vi "RefStruct_CONVERT.vi"(1 "RefStruct":T12={"RefNormal"={"Mode"=0, "Fliter"=1, "AccCode"=0, "AccMask"=0, "kBaudRate"=0, "Timing0"=0, "Timing1"=0, "CANRX_EN"=0, "UARTBAUD"=0}, "Reserved"=0, "BaudType"={"Baud"=0, "SJW"=1, "BRP"=1, "SAM"=0, "PHSEG2_SEL"=0, "PRSEG"=1, "PHSEG1"=1, "PHSEG2"=1}} {"RefNormal"."kBaudRate" items=["SelfDefine", "5 kbps", "10 kbps", "20 kbps", "40 kbps", "50 kbps", "80 kbps", "100 kbps", "125 kbps", "200 kbps", "250 kbps", "400 kbps", "500 kbps", "666 kbps", "800 kbps", "1000 kbps", "33.33 kbps", "66.66 kbps", "83.33 kbps"]; "RefNormal"."AccMask" format="%x"; "RefNormal"."AccCode" format="%x"; "RefNormal"."Fliter" items=["接收所有类型"=1, "只接收标准帧"=2, "只接收扩展帧"=3]; "RefNormal"."Mode" items=["正常工作", "仅侦听模式", "自测模式（环回）"]; "BaudType"."PHSEG2" items=["CAN_BIT_1TQ"=1, "CAN_BIT_2TQ"=2, "CAN_BIT_3TQ"=3, "CAN_BIT_4TQ"=4, "CAN_BIT_5TQ"=5, "CAN_BIT_6TQ"=6, "CAN_BIT_7TQ"=7, "CAN_BIT_8TQ"=8]; "BaudType"."PHSEG1" items=["CAN_BIT_1TQ"=1, "CAN_BIT_2TQ"=2, "CAN_BIT_3TQ"=3, "CAN_BIT_4TQ"=4, "CAN_BIT_5TQ"=5, "CAN_BIT_6TQ"=6, "CAN_BIT_7TQ"=7, "CAN_BIT_8TQ"=8]; "BaudType"."PRSEG" items=["CAN_BIT_1TQ"=1, "CAN_BIT_2TQ"=2, "CAN_BIT_3TQ"=3, "CAN_BIT_4TQ"=4, "CAN_BIT_5TQ"=5, "CAN_BIT_6TQ"=6, "CAN_BIT_7TQ"=7, "CAN_BIT_8TQ"=8]; "BaudType"."PHSEG2_SEL" items=["由相位缓冲段1时间决定", "可编程"]; "BaudType"."SAM" items=["采样一次", "采样三次"]; "BaudType"."BRP" items=["1"=1, "2"=2, "3"=3, "4"=4, "5"=5, "6"=6, "7"=7, "8"=8, "9"=9, "10"=10, "11"=11, "12"=12, "13"=13, "14"=14, "15"=15, "16"=16, "17"=17, "18"=18, "19"=19, "20"=20, "21"=21, "22"=22, "23"=23, "24"=24, "25"=25, "26"=26, "27"=27, "28"=28, "29"=29, "30"=30, "31"=31, "32"=32, "33"=33, "34"=34, "35"=35, "36"=36, "37"=37, "38"=38, "39"=39, "40"=40, "41"=41, "42"=42, "43"=43, "44"=44, "45"=45, "46"=46, "47"=47, "48"=48, "49"=49, "50"=50, "51"=51, "52"=52, "53"=53, "54"=54, "55"=55, "56"=56, "57"=57, "58"=58, "59"=59, "60"=60, "61"=61, "62"=62, "63"=63, "64"=64]; "BaudType"."SJW" items=["1TQ"=1, "2TQ"=2, "3TQ"=3, "4TQ"=4]}) -> (0 "RefStruct_1":T1={"Mode"=0, "Fliter"=1, "ACR 0"=0, "ACR 1"=0, "ACR 2"=0, "ACR 3"=0, "AMR 0"=0, "AMR 1"=0, "AMR 2"=0, "AMR 3"=0, "kBaudRate"=0, "Timing 0"=0, "Timing 1"=0, "CANRX_EN"=0, "UARTBAUD"=0, "Reserved"=0, "Baud 0"=0, "Baud 1"=0, "Baud 2"=0, "Baud 3"=0, "SJW"=1, "BRP"=1, "SAM"=0, "PHSEG2_SEL"=0, "PRSEG"=1, "PHSEG1"=1, "PHSEG2"=1} {"PHSEG2" items=["CAN_BIT_1TQ"=1, "CAN_BIT_2TQ"=2, "CAN_BIT_3TQ"=3, "CAN_BIT_4TQ"=4, "CAN_BIT_5TQ"=5, "CAN_BIT_6TQ"=6, "CAN_BIT_7TQ"=7, "CAN_BIT_8TQ"=8]; "PHSEG1" items=["CAN_BIT_1TQ"=1, "CAN_BIT_2TQ"=2, "CAN_BIT_3TQ"=3, "CAN_BIT_4TQ"=4, "CAN_BIT_5TQ"=5, "CAN_BIT_6TQ"=6, "CAN_BIT_7TQ"=7, "CAN_BIT_8TQ"=8]; "PRSEG" items=["CAN_BIT_1TQ"=1, "CAN_BIT_2TQ"=2, "CAN_BIT_3TQ"=3, "CAN_BIT_4TQ"=4, "CAN_BIT_5TQ"=5, "CAN_BIT_6TQ"=6, "CAN_BIT_7TQ"=7, "CAN_BIT_8TQ"=8]; "PHSEG2_SEL" items=["由相位缓冲段1时间决定", "可编程"]; "SAM" items=["采样一次", "采样三次"]; "BRP" items=["1"=1, "2"=2, "3"=3, "4"=4, "5"=5, "6"=6, "7"=7, "8"=8, "9"=9, "10"=10, "11"=11, "12"=12, "13"=13, "14"=14, "15"=15, "16"=16, "17"=17, "18"=18, "19"=19, "20"=20, "21"=21, "22"=22, "23"=23, "24"=24, "25"=25, "26"=26, "27"=27, "28"=28, "29"=29, "30"=30, "31"=31, "32"=32, "33"=33, "34"=34, "35"=35, "36"=36, "37"=37, "38"=38, "39"=39, "40"=40, "41"=41, "42"=42, "43"=43, "44"=44, "45"=45, "46"=46, "47"=47, "48"=48, "49"=49, "50"=50, "51"=51, "52"=52, "53"=53, "54"=54, "55"=55, "56"=56, "57"=57, "58"=58, "59"=59, "60"=60, "61"=61, "62"=62, "63"=63, "64"=64]; "SJW" items=["1TQ"=1, "2TQ"=2, "3TQ"=3, "4TQ"=4]; "kBaudRate" items=["SelfDefine", "5 kbps", "10 kbps", "20 kbps", "40 kbps", "50 kbps", "80 kbps", "100 kbps", "125 kbps", "200 kbps", "250 kbps", "400 kbps", "500 kbps", "666 kbps", "800 kbps", "1000 kbps", "33.33 kbps", "66.66 kbps", "83.33 kbps"]; "Fliter" items=["接收所有类型"=1, "只接收标准帧"=2, "只接收扩展帧"=3]; "Mode" items=["正常工作", "仅侦听模式", "自测模式（环回）"]})   [LabVIEW 2018, in "ControlCan.lvlib"]
uses:
  ControlCan.lvlib
  RefStruct.ctl
  RefNormal.ctl
  Mode.ctl
  Fliter.ctl
  kBaudRate.ctl
  BaudType.ctl
  SJW.ctl
  BRP.ctl
  SAM.ctl
  PHSEG2_SEL.ctl
  PRSEG.ctl
  PHSEG1.ctl
  PHSEG2.ctl
  RefStruct_1.ctl
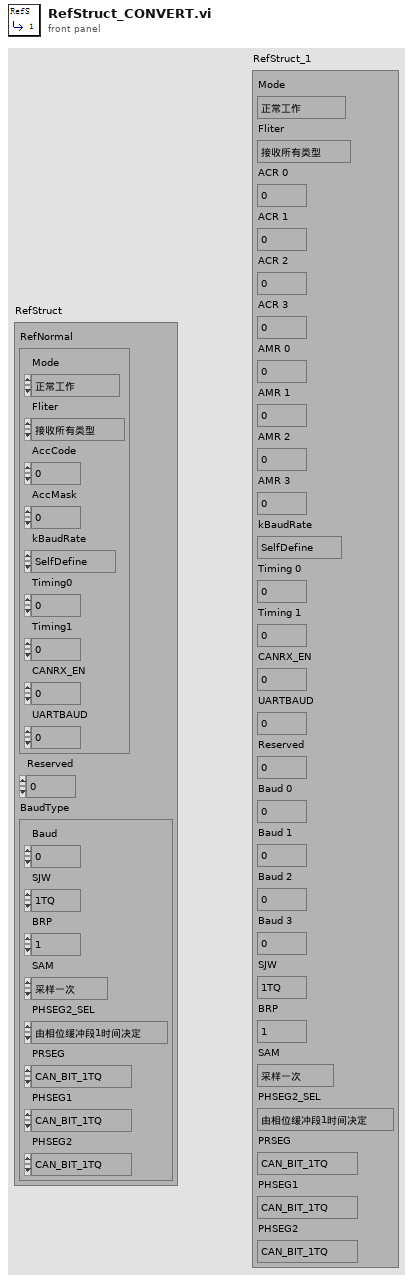
[diagram p1: front panel]
types:
  T1 = typedef "ControlCAN.lvlib/RefStruct_1.ctl" = cluster{"Mode":T2, "Fliter":T3, "ACR 0":u8, "ACR 1":u8, "ACR 2":u8, "ACR 3":u8, "AMR 0":u8, "AMR 1":u8, "AMR 2":u8, "AMR 3":u8, "kBaudRate":T4, "Timing 0":u8, "Timing 1":u8, "CANRX_EN":u8, "UARTBAUD":u8, "Reserved":u8, "Baud 0":u8, "Baud 1":u8, "Baud 2":u8, "Baud 3":u8, "SJW":T5, "BRP":T6, "SAM":T7, "PHSEG2_SEL":T8, "PRSEG":T9, "PHSEG1":T10, "PHSEG2":T11}
  T2 = typedef "ControlCAN.lvlib/Mode.ctl" = u8
  T3 = typedef "ControlCAN.lvlib/Fliter.ctl" = u8
  T4 = typedef "ControlCAN.lvlib/kBaudRate.ctl" = u8
  T5 = typedef "ControlCAN.lvlib/SJW.ctl" = u8
  T6 = typedef "ControlCAN.lvlib/BRP.ctl" = u8
  T7 = typedef "ControlCAN.lvlib/SAM.ctl" = u8
  T8 = typedef "ControlCAN.lvlib/PHSEG2_SEL.ctl" = u8
  T9 = typedef "ControlCAN.lvlib/PRSEG.ctl" = u8
  T10 = typedef "ControlCAN.lvlib/PHSEG1.ctl" = u8
  T11 = typedef "ControlCAN.lvlib/PHSEG2.ctl" = u8
  T12 = typedef "ControlCAN.lvlib/RefStruct.ctl" = cluster{"RefNormal":T13, "Reserved":u8, "BaudType":T14}
  T13 = typedef "ControlCAN.lvlib/RefNormal.ctl" = cluster{"Mode":T2, "Fliter":T3, "AccCode":u32, "AccMask":u32, "kBaudRate":T4, "Timing0":u8, "Timing1":u8, "CANRX_EN":u8, "UARTBAUD":u8}
  T14 = typedef "ControlCAN.lvlib/BaudType.ctl" = cluster{"Baud":u32, "SJW":T5, "BRP":T6, "SAM":T7, "PHSEG2_SEL":T8, "PRSEG":T9, "PHSEG1":T10, "PHSEG2":T11}
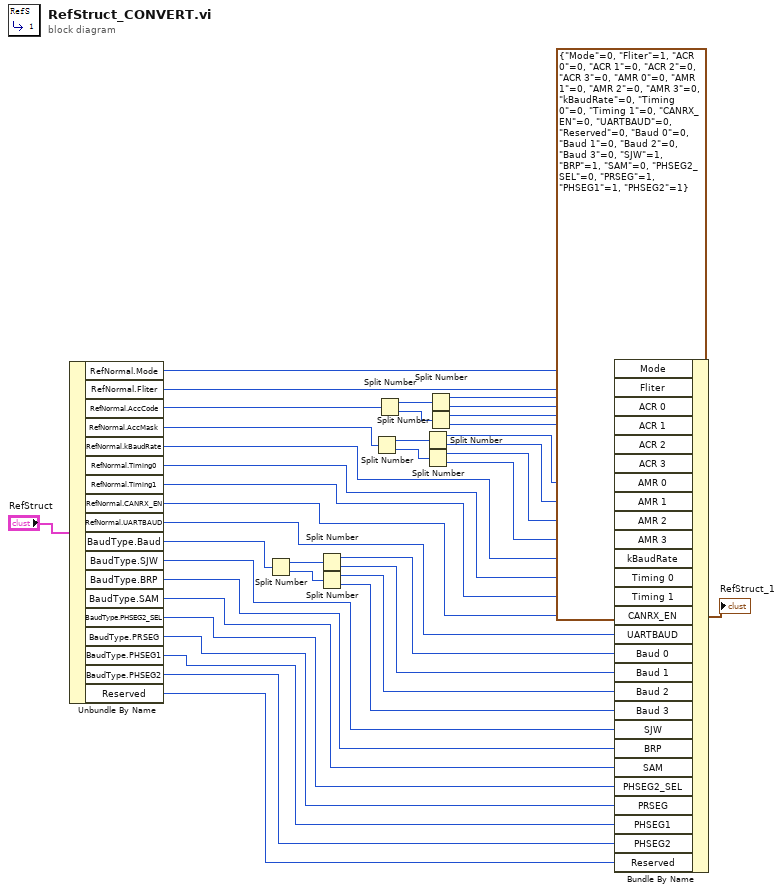
[diagram p0: block diagram]
diagram:
  n1 = Unbundle By Name("RefStruct") -> ("RefNormal.Mode"=w37:T2, "RefNormal.Fliter"=w36:T3, "RefNormal.AccCode"=w35:u32, "RefNormal.AccMask"=w26:u32, "RefNormal.kBaudRate"=w21:T4, "RefNormal.Timing0"=w20:u8, "RefNormal.Timing1"=w19:u8, "RefNormal.CANRX_EN"=w18:u8, "RefNormal.UARTBAUD"=w17:u8, "BaudType.Baud"=w14:u32, "BaudType.SJW"=w9:T5, "BaudType.BRP"=w8:T6, "BaudType.SAM"=w7:T7, "BaudType.PHSEG2_SEL"=w6:T8, "BaudType.PRSEG"=w5:T9, "BaudType.PHSEG1"=w4:T10, "BaudType.PHSEG2"=w3:T11, "Reserved"=w1:u8)
  n2 = Split Number(x=w14) -> (hi(x)=w16:u16, lo(x)=w15:u16)
  n3 = Split Number(x=w16) -> (hi(x)=w13:u8, lo(x)=w12:u8)
  n4 = Split Number(x=w15) -> (hi(x)=w11:u8, lo(x)=w10:u8)
  n5 = Split Number(x=w26) -> (hi(x)=w28:u16, lo(x)=w27:u16)
  n6 = Split Number(x=w35) -> (hi(x)=w34:u16, lo(x)=w33:u16)
  n7 = Split Number(x=w28) -> (hi(x)=w25:u8, lo(x)=w24:u8)
  n8 = Split Number(x=w27) -> (hi(x)=w23:u8, lo(x)=w22:u8)
  n9 = Split Number(x=w34) -> (hi(x)=w32:u8, lo(x)=w31:u8)
  n10 = Split Number(x=w33) -> (hi(x)=w30:u8, lo(x)=w29:u8)
  n11 = Bundle By Name(cluster=T1 {"Mode"=0, "Fliter"=1, "ACR 0"=0, "ACR 1"=0, "ACR 2"=0, "ACR 3"=0, "AMR 0"=0, "AMR 1"=0, "AMR 2"=0, "AMR 3"=0, "kBaudRate"=0, "Timing 0"=0, "Timing 1"=0, "CANRX_EN"=0, "UARTBAUD"=0, "Reserved"=0, "Baud 0"=0, "Baud 1"=0, "Baud 2"=0, "Baud 3"=0, "SJW"=1, "BRP"=1, "SAM"=0, "PHSEG2_SEL"=0, "PRSEG"=1, "PHSEG1"=1, "PHSEG2"=1} ("RefStruct_1"), "Mode"=w37, "Fliter"=w36, "ACR 0"=w32, "ACR 1"=w31, "ACR 2"=w30, "ACR 3"=w29, "AMR 0"=w25, "AMR 1"=w24, "AMR 2"=w23, "AMR 3"=w22, "kBaudRate"=w21, "Timing 0"=w20, "Timing 1"=w19, "CANRX_EN"=w18, "UARTBAUD"=w17, "Baud 0"=w13, "Baud 1"=w12, "Baud 2"=w11, "Baud 3"=w10, "SJW"=w9, "BRP"=w8, "SAM"=w7, "PHSEG2_SEL"=w6, "PRSEG"=w5, "PHSEG1"=w4, "PHSEG2"=w3, "Reserved"=w1) -> (→"RefStruct_1":T1)
